vi "phase_maps_to_pixel_difference.vi"(10 "dist phase map":i32[][](array[numeric]), 11 "oirg phase map":i32[][](array[numeric])) -> (3 "displacement map":i32[][](array[numeric]))   [LabVIEW 2011]
doc: "The input array must be unwrapped phase maps, that are normalize to the same span (i.e. 0 to 255) and where the masked pixels are 0."
uses:
  global_vars.vi
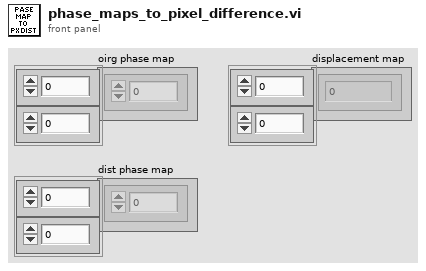
[diagram p1: front panel]
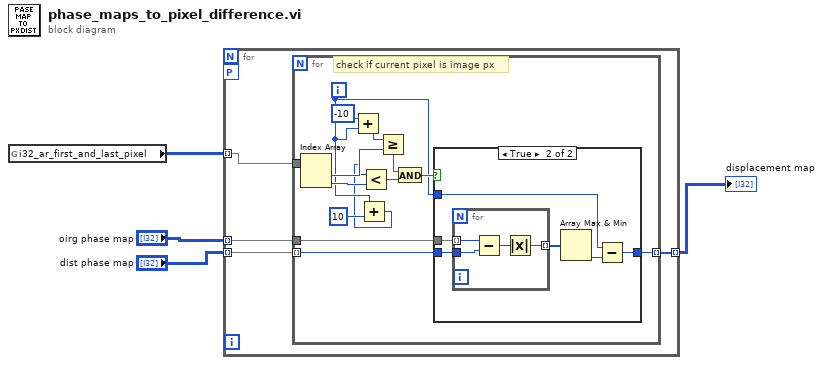
[diagram p0: block diagram]
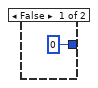
[diagram p2: hidden frame]
diagram:
  n1 = global read "global_vars.vi" "i32_ar_first_and_last_pixel"() -> (w1:i32[][])
  n2 = for {
    tunnel: "dist phase map" -> [w8] mode=indexing
    tunnel: "oirg phase map" -> [w7] mode=indexing
    workers-P: _ -> [_]
    tunnel: [w6] -> w4 mode=indexing
    tunnel: w1 -> [w5] mode=indexing
    n3 = for {
      tunnel: w8 -> [w22] mode=indexing
      tunnel: [w21] -> w6 mode=indexing
      tunnel: w7 -> [w20]
      tunnel: w5 -> [w15]
      i -> [w11]
      # "check if current pixel is image px"
      n4 = Index Array(array=w15) -> (element #1=w18:i32, element #2=w19:i32)  [unwired: 2 in]
      n5 = Add(x=-10, y=w11) -> (x+y=w13:i32)
      n6 = Add(x=w11, y=10) -> (x+y=w9:i32)
      n7 = Less?(x=w9, y=w19) -> (x < y?=w16:bool)
      n8 = Greater Or Equal?(x=w13, y=w18) -> (x >= y?=w17:bool)
      n9 = And(x=w17, y=w16) -> (x .and. y?=w14:bool)
      n10 = case shown="True" w14 {
        tunnel: w22 -> [_ w29]
        tunnel: [0 w24] -> w21
        tunnel: w20 -> [_ w26]
        tunnel: w11 -> [_ w25]
        frame False {
        }
        frame True {
          n11 = for {
            tunnel: w26 -> [w33] mode=indexing
            tunnel: w29 -> [w32]
            tunnel: [w31] -> w28 mode=indexing
            n12 = Subtract(x=w33, y=w32) -> (x-y=w30:i32)
            n13 = Absolute Value(x=w30) -> (abs(x)=w31:i32)
          }
          n14 = Array Max & Min(array=w28) -> (min index (indices)=w27:i32)  [unwired: 3 out]
          n15 = Subtract(x=w25, y=w27) -> (x-y=w24:i32)
        }
      }
    }
  }
  "displacement map" <- w4
